vi "PWM Configure.vi"(6 "period [ms]":u32=1000 min=2 max=500000, 7 "active LOW":u8, 8 "error in (no error)":errorcluster, 9 "channel B duty":sgl, 10 "channel A duty":sgl, 11 "Task in":refnum<class "PWM.lvclass">) -> (0 "error out":errorcluster, 3 "Task out":refnum<class "PWM.lvclass">)   [LabVIEW 2009, in "MicroDAQ.lvlib" / "PWM.lvclass"]
uses:
  <instrlib>/MicroDAQ/Channel/PWM/PWM.lvclass
  <instrlib>/MicroDAQ/Channel/PWM/PWM.lvclass/PWM.ctl
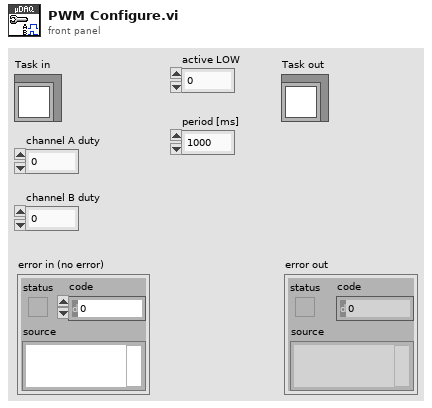
[diagram p1: front panel]
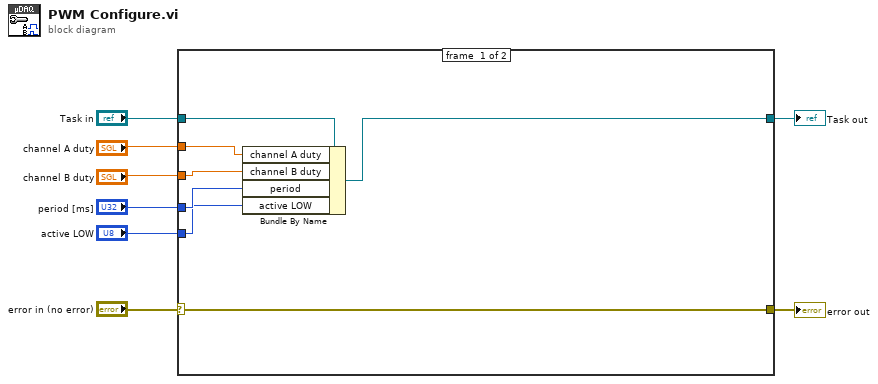
[diagram p0: block diagram]
diagram:
  n1 = case shown="No Error" "error in (no error)" {
    selector: "error in (no error)" -> [w12 w16]
    tunnel: [w12 w16] -> w7
    tunnel: "Task in" -> [w15 w17]
    tunnel: [w14 w17] -> w5
    tunnel: "period [ms]" -> [w13 _]
    tunnel: "active LOW" -> [w11 _]
    tunnel: "channel A duty" -> [w10 _]
    tunnel: "channel B duty" -> [w9 _]
    frame #0 {
      n2 = Bundle By Name(cluster=w15, "channel A duty"=w10, "channel B duty"=w9, "period"=w13, "active LOW"=w11) -> (w14:refnum<class "PWM.lvclass">)
    }
    frame #1 {
    }
  }
  "error out" <- w7
  "Task out" <- w5
